vi "giveAirJuicer.vi"(6 "seconds since 1Jan1904 2":timestamp, 8 "error in (no error)":errorcluster, 9 "IRI":dbl, 10 "Window Number (0...15)":i32, 11 "Juicer in":refnum<class "Juicer.lvclass">) -> (0 "error out":errorcluster, 1 "seconds since 1Jan1904":timestamp, 3 "Juicer out":refnum<class "Juicer.lvclass">)   [LabVIEW 2014, in "Juicer.lvclass"]
uses:
  Juicer.lvclass
  Juicer.lvclass/Juicer.ctl
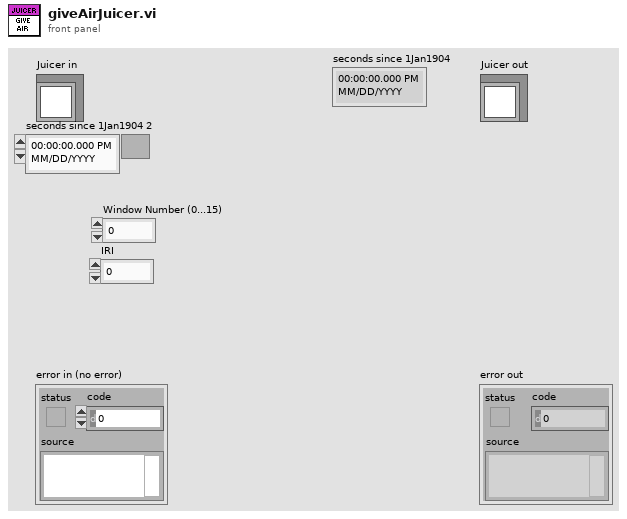
[diagram p1: front panel]
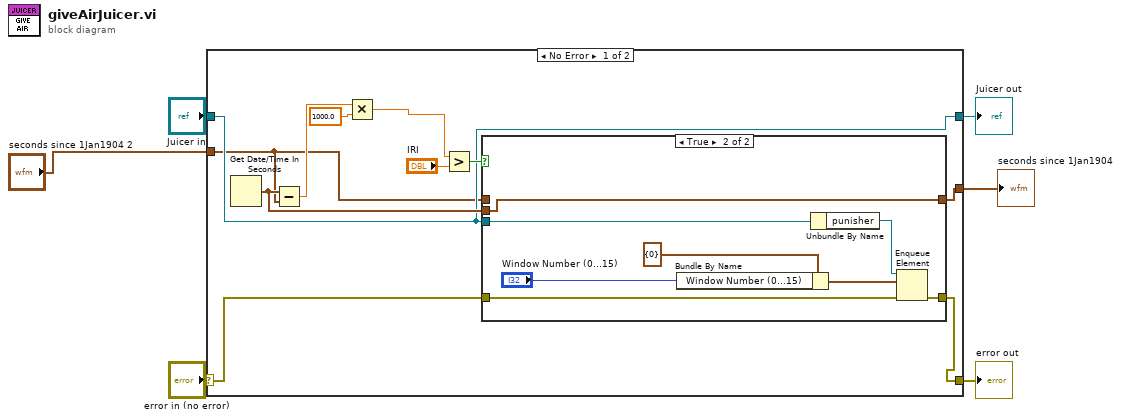
[diagram p0: block diagram]
diagram:
  n1 = case shown="No Error" "error in (no error)" {
    selector: "error in (no error)" -> [w11 w30]
    tunnel: [w12 w30] -> w5
    tunnel: [w10 w29] -> w3
    tunnel: "Juicer in" -> [w10 w29]
    tunnel: "seconds since 1Jan1904 2" -> [w9 w28]
    tunnel: [w8 w28] -> w1
    frame No Error {
      n2 = Get Date/Time In Seconds() -> (seconds since 1Jan1904=w17:timestamp)
      n3 = Subtract(x=w17, y=w9) -> (x-y=w14:dbl)
      n4 = Multiply(x=w14, y=1000.0) -> (x*y=w7:dbl)
      n5 = Greater?(x=w7, y="IRI") -> (0:w15:bool)
      n6 = case shown="True" w15 {
        tunnel: w10 -> [_ w27]
        tunnel: w11 -> [w18 w22]
        tunnel: [w18 w21] -> w12
        tunnel: [w19 w20] -> w8
        tunnel: w9 -> [w19 _]
        tunnel: w17 -> [_ w20]
        frame False {
        }
        frame True {
          n7 = Bundle By Name(cluster=cluster{"Window Number (0...15)":i32} {"Window Number (0...15)"=0} ("element"), "Window Number (0...15)"="Window Number (0...15)") -> (w24:cluster{"Window Number (0...15)":i32})
          n8 = Unbundle By Name(w27) -> ("punisher"=w26:refnum<queue>)
          n9 = Enqueue Element(queue=w26, element=w24, error in (no error)=w22) -> (error out=w21:errorcluster)  [unwired: 1 in, 2 out]
        }
      }
    }
    frame Error {
    }
  }
  "error out" <- w5
  "Juicer out" <- w3
  "seconds since 1Jan1904" <- w1
